vi "MDTM Data to TimeStamp.vi"(8 "error in (no error)":errorcluster, 10 "MDTM Data":string, 11 "FTP in":refnum<class "FTP.lvclass">) -> (0 "error out":errorcluster, 2 "time stamp":timestamp, 3 "FTP out":refnum<class "FTP.lvclass">)   [LabVIEW 2017, in "FTP_UpgradeCSMF.lvlib" / "FTP.lvclass"]
uses:
  FTP.lvclass
  <vilib>/Utility/miscctls.llb/LVDateTimeRec.ctl
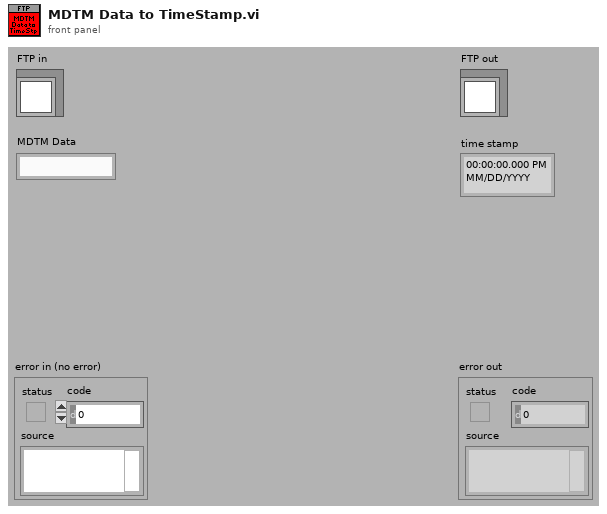
[diagram p1: front panel]
types:
  T1 = typedef "LVDateTimeRec.ctl" = cluster{"fractional second":dbl, "second":i32, "minute":i32, "hour":i32, "day of month":i32, "month":i32, "year":i32, "day of week":i32, "day of year":i32, "DST":i32}
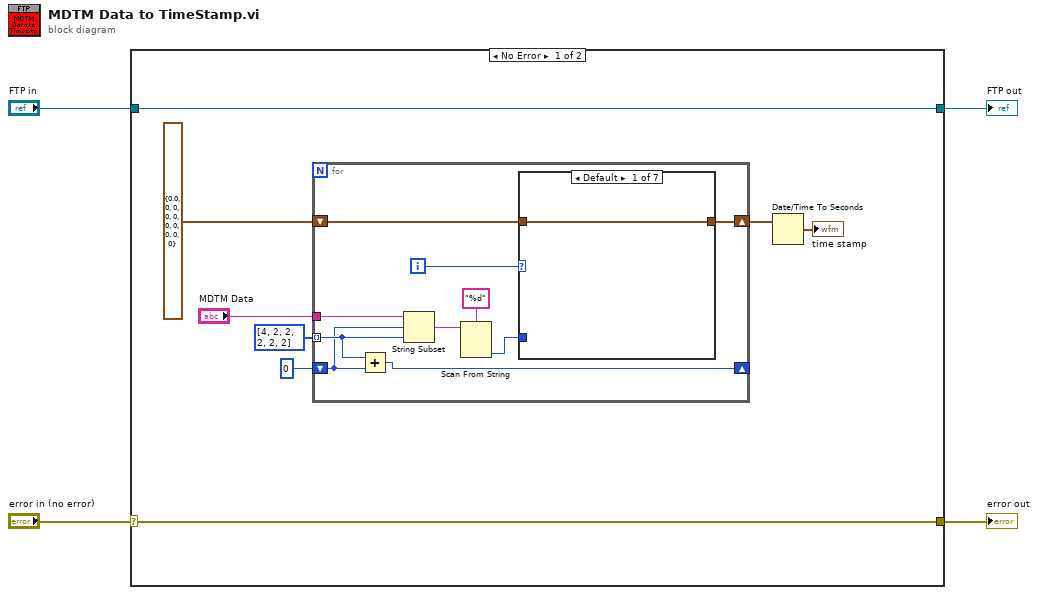
[diagram p0: block diagram]
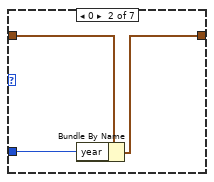
[diagram p2: hidden frame]
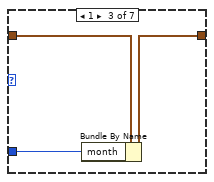
[diagram p3: hidden frame]
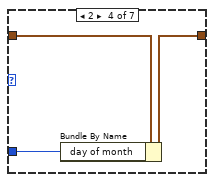
[diagram p4: hidden frame]
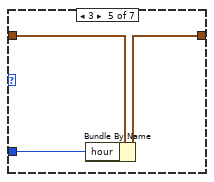
[diagram p5: hidden frame]
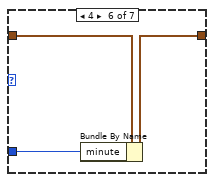
[diagram p6: hidden frame]
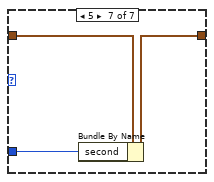
[diagram p7: hidden frame]
diagram:
  n1 = case shown="No Error" "error in (no error)" {
    selector: "error in (no error)" -> [w11 w43]
    tunnel: [w11 w43] -> w3
    tunnel: [w12 w42] -> w1
    tunnel: "FTP in" -> [w12 w42]
    frame No Error {
      n2 = for {
        tunnel: "MDTM Data" -> [w22]
        tunnel: i32[] [4, 2, 2, 2, 2, 2] -> [w21] mode=indexing
        shift-right: [w19] -> _
        shift-left: 0 -> [w20]
        shift-right: [w13] -> w6
        shift-left: T1 {"fractional second"=0.0, "second"=0, "minute"=0, "hour"=0, "day of month"=0, "month"=0, "year"=0, "day of week"=0, "day of year"=0, "DST"=0} ("date time rec") -> [w17]
        i -> [w18]
        n3 = Add(x=w21, y=w20) -> (x+y=w19:i32)
        n4 = String Subset(string=w22, offset (0)=w20, length (rest)=w21) -> (substring=w15:string)
        n5 = Scan From String(format string="%d", input string=w15) -> (output 1=w14:i32)  [unwired: 3 in, 3 out]
        n6 = case shown="Default" w18 {
          tunnel: w17 -> [w23 w26 w29 w32 w35 w38 w41]
          tunnel: w14 -> [_ w25 w28 w31 w34 w37 w40]
          tunnel: [w23 w24 w27 w30 w33 w36 w39] -> w13
          frame Default {
          }
          frame 0 {
            n7 = Bundle By Name(cluster=w26, "year"=w25) -> (w24:T1)
          }
          frame 1 {
            n8 = Bundle By Name(cluster=w29, "month"=w28) -> (w27:T1)
          }
          frame 2 {
            n9 = Bundle By Name(cluster=w32, "day of month"=w31) -> (w30:T1)
          }
          frame 3 {
            n10 = Bundle By Name(cluster=w35, "hour"=w34) -> (w33:T1)
          }
          frame 4 {
            n11 = Bundle By Name(cluster=w38, "minute"=w37) -> (w36:T1)
          }
          frame 5 {
            n12 = Bundle By Name(cluster=w41, "second"=w40) -> (w39:T1)
          }
        }
      }
      n13 = Date/Time To Seconds(2:w6) -> (0:→"time stamp":timestamp)  [unwired: 1 in]
    }
    frame Error {
    }
  }
  "error out" <- w3
  "FTP out" <- w1
